vi "Cryo-Con Set Manual Heater Value.vi"() -> ()   [LabVIEW 2016]
panel:
  in  "Set heat %":dbl
  out "resulting string":string
  out "VISA Resource Name Out":refnum<visa-resource-name>
  in  "VISA Resource Name 2":refnum<visa-resource-name>
  out "error out":errorcluster
  in  "error in (no error)":errorcluster
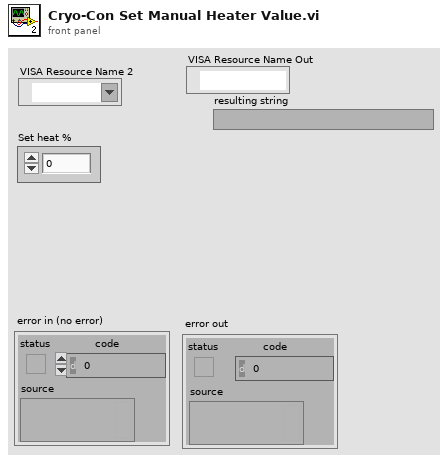
[diagram p1: front panel]
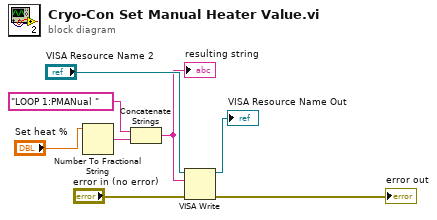
[diagram p0: block diagram]
diagram:
  n1 = Number To Fractional String(number="Set heat %") -> (F-format string=w2:string)  [unwired: 3 in]
  n2 = Concatenate Strings("LOOP 1:PMANual " ("format string"), w2) -> (w4:string)
  "resulting string" <- w4
  n3 = VISA Write(VISA resource name="VISA Resource Name 2", write buffer=w4, error in (no error)="error in (no error)") -> (VISA resource name out=→"VISA Resource Name Out":refnum<visa-resource-name>, error out=→"error out":errorcluster)  [unwired: 1 out]
